vi "Optical Encoder.vi"(2 "Stop":bool, 3 "B Input Terminal":tag, 4 "A Input Terminal":tag, 5 "Encorder Counter":tag) -> (0 "Position (degrees)":dbl format="%0.2f", 1 "RPM":dbl)   [LabVIEW 2017]
uses:
  <vilib>/DAQmx/read.llb/DAQmx Read (Counter DBL 1Chan 1Samp).vi
  <vilib>/DAQmx/create/channels.llb/DAQmx Create Channel (CI-Position-Angular Encoder).vi
  <vilib>/DAQmx/miscellaneous.llb/DAQmx Fill In Error Info.vi
  <resource>/objmgr/daqmx.rc
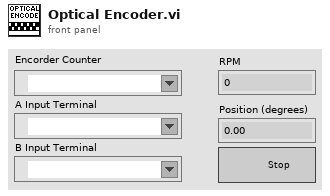
[diagram p1: front panel]
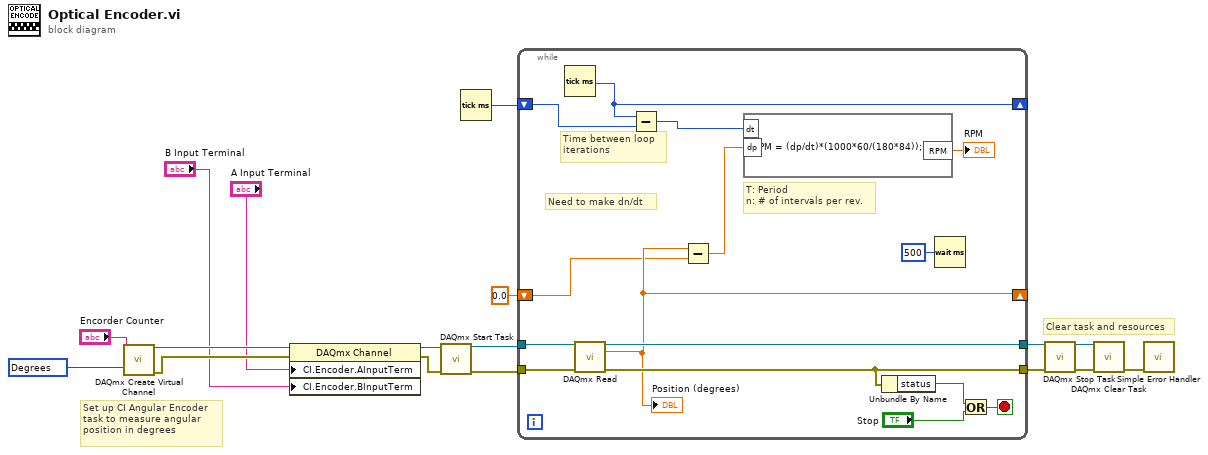
[diagram p0: block diagram]
diagram:
  w8 = 10146 items=["Degrees"=10146, "Radians"=10273, "Ticks"=10304, "From Custom Scale"=10065] ("units")
  # "Clear task and resources"
  # "Set up CI Angular Encoder\ntask to measure angular\nposition in degrees"
  n1 = call-poly <vilib>:"DAQmx Create Virtual Channel.vi"("counter"="Encorder Counter", "units"=w8) -> ("task out"=w16:refnum<k21>, "error out"=w15:errorcluster)  [unwired: 12 in]
  n2 = property class="DAQmx Channel"(reference=w16, error in=w15, "CI.Encoder.AInputTerm"="A Input Terminal", "CI.Encoder.BInputTerm"="B Input Terminal") -> (reference out=w12:refnum<k21>, error out=w11:errorcluster)
  n3 = call <vilib>:"DAQmx Start Task.vi"("task/channels in"=w12, "error in"=w11) -> ("task out"=w10:refnum<k21>, "error out"=w9:errorcluster)  [unwired: 12 in]
  n4 = Tick Count (ms)() -> (millisecond timer value=w2:u32)
  n5 = while {
    tunnel: w10 -> [w32]
    tunnel: w9 -> [w31]
    tunnel: [w28] -> w6
    tunnel: [w29] -> w7
    shift-right: [w24] -> _
    shift-left: w2 -> [w25]
    shift-right: [w21] -> _
    shift-left: 0.0 ("data") -> [w20]
    stop <- w30 stop-if-true
    # "Need to make dn/dt"
    # "Time between loop\niterations"
    # "T: Period\nn: # of intervals per rev."
    n6 = Tick Count (ms)() -> (millisecond timer value=w24:u32)
    n7 = call-poly <vilib>:"DAQmx Read.vi"("task/channels in"=w32, "error in"=w31) -> ("task out"=w29:refnum<k21>, "data"=w21:dbl, "error out"=w28:errorcluster)  [unwired: 11 in]
    "Position (degrees)" <- w21
    n8 = Subtract(x=w24, y=w25) -> (x-y=w23:u32)
    n9 = Subtract(x=w21, y=w20) -> (x-y=w19:dbl)
    n10 = formula code="RPM = (dp/dt)*(1000*60/(180*84));"("dt"=w23, "dp"=w19) -> ("RPM"=→"RPM":dbl)
    n11 = Unbundle By Name(w28) -> ("status"=w27:bool)
    n12 = Wait (ms)(milliseconds to wait=u32 500) -> ()  [unwired: 1 out]
    n13 = Or(x=w27, y="Stop") -> (x .or. y?=w30:bool)
  }
  n14 = call <vilib>:"DAQmx Stop Task.vi"("task/channels in"=w7, "error in"=w6) -> ("task out"=w5:refnum<k21>, "error out"=w4:errorcluster)  [unwired: 12 in]
  n15 = call <vilib>:"DAQmx Clear Task.vi"("task in"=w5, "error in"=w4) -> ("error out"=w3:errorcluster)  [unwired: 13 in]
  n16 = call <vilib>:"Simple Error Handler.vi"("error in (no error)"=w3) -> ()  [unwired: 4 in, 5 out]
